vi "Parse NT Data.vi"(10 "Cluster":T1, 11 "TCP Network Connection in":refnum<k5>) -> (1 "Size":i32, 3 "Field Value Out":T2)   [LabVIEW 2017]
uses:
  <vilib>/Rock Robotics/Network Tables/Field Data.ctl
  <vilib>/Rock Robotics/Network Tables/Field Type.ctl
  <vilib>/Rock Robotics/Network Tables/Sequence.ctl
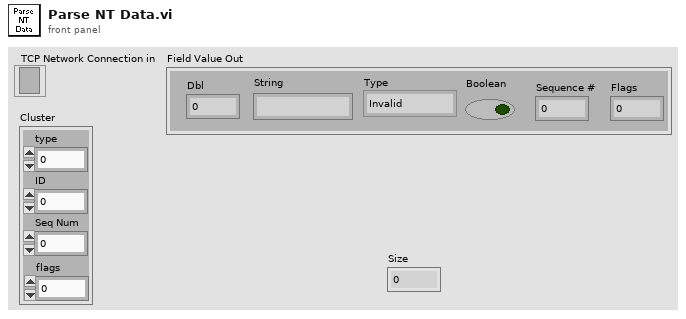
[diagram p1: front panel]
types:
  T1 = cluster{"type":u8, "ID":u16, "Seq Num":u16, "flags":u8}
  T2 = typedef "Field Data.ctl" = cluster{"Dbl":dbl, "String":string, "Type":T3, "Boolean":bool, "Sequence #":T4, "Flags":u8}
  T3 = typedef "Field Type.ctl" = enum8{"Invalid", "Bool", "Numeric", "String", "Raw", "Boolean Array", "Numeric Array", "String Array", "RPC"}
  T4 = typedef "Sequence.ctl" = u16
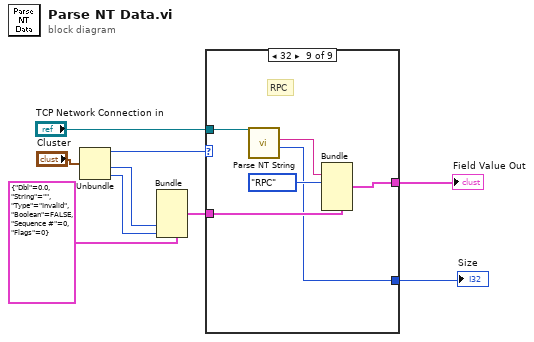
[diagram p0: block diagram]
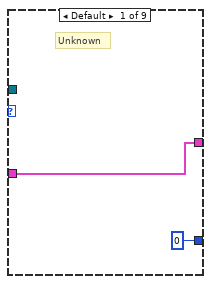
[diagram p2: hidden frame]
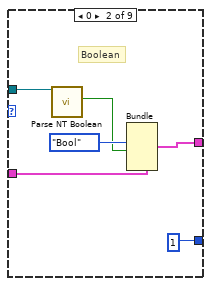
[diagram p3: hidden frame]
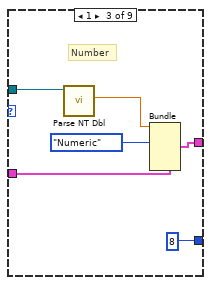
[diagram p4: hidden frame]
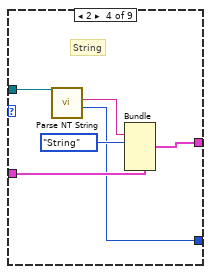
[diagram p5: hidden frame]
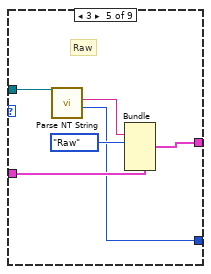
[diagram p6: hidden frame]
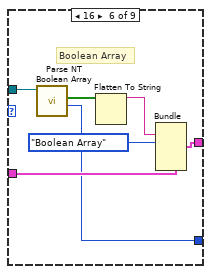
[diagram p7: hidden frame]
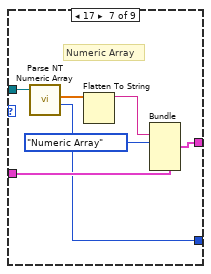
[diagram p8: hidden frame]
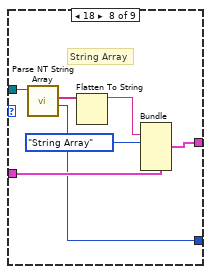
[diagram p9: hidden frame]
diagram:
  n1 = Unbundle("Cluster") -> ("type"=w7:u8, "Seq Num"=w3:u16, "flags"=w1:u8)  [unwired: 1 out]
  n2 = Bundle(cluster=T2 {"Dbl"=0.0, "String"="", "Type"=enum."Invalid", "Boolean"=FALSE, "Sequence #"=0, "Flags"=0} ("Field Value Out"), "Sequence #"=w3, "Flags"=w1) -> (w4:T2)  [unwired: 4 in]
  n3 = case shown="32" w7 {
    tunnel: "TCP Network Connection in" -> [_ w17 w23 w29 w35 w42 w49 w56 w62]
    tunnel: w4 -> [w11 w16 w21 w27 w33 w40 w47 w54 w60]
    tunnel: [w11 w13 w19 w25 w31 w39 w46 w53 w58] -> w9
    tunnel: [0 1 8 w24 w30 w36 w43 w50 w57] -> w2
    frame Default {
      # "Unknown"
    }
    frame 0 {
      # "Boolean"
      n4 = call <vilib>:"Parse NT Boolean.vi"("TCP Network Connection in"=w17) -> ("Boolean"=w14:bool)  [unwired: 9 in, 1 out]
      n5 = Bundle(cluster=w16, "Type"=Field_Type."Bool", "Boolean"=w14) -> (w13:T2)  [unwired: 4 in]
    }
    frame 1 {
      # "Number"
      n6 = call <vilib>:"Parse NT Dbl.vi"("TCP Network Connection in"=w23) -> ("Double"=w20:dbl)  [unwired: 9 in, 1 out]
      n7 = Bundle(cluster=w21, "Dbl"=w20, "Type"=Field_Type."Numeric") -> (w19:T2)  [unwired: 4 in]
    }
    frame 2 {
      # "String"
      n8 = call <vilib>:"Parse NT String.vi"("TCP Network Connection in"=w29) -> ("Size"=w24:i32, "String"=w26:string)  [unwired: 8 in, 1 out]
      n9 = Bundle(cluster=w27, "String"=w26, "Type"=Field_Type."String") -> (w25:T2)  [unwired: 4 in]
    }
    frame 3 {
      # "Raw"
      n10 = call <vilib>:"Parse NT String.vi"("TCP Network Connection in"=w35) -> ("Size"=w30:i32, "String"=w32:string)  [unwired: 8 in, 1 out]
      n11 = Bundle(cluster=w33, "String"=w32, "Type"=Field_Type."Raw") -> (w31:T2)  [unwired: 4 in]
    }
    frame 16 {
      # "Boolean Array"
      n12 = call <vilib>:"Parse NT Boolean Array.vi"("TCP Network Connection in"=w42) -> ("Size"=w36:i32, "Boolean Array"=w38:bool[])  [unwired: 7 in, 2 out]
      n13 = Flatten To String(anything=w38) -> (data string=w37:string)  [unwired: 3 in, 2 out]
      n14 = Bundle(cluster=w40, "String"=w37, "Type"=Field_Type."Boolean Array") -> (w39:T2)  [unwired: 4 in]
    }
    frame 17 {
      # "Numeric Array"
      n15 = call <vilib>:"Parse NT Numeric Array.vi"("TCP Network Connection in"=w49) -> ("Size"=w43:i32, "Numeric Array"=w45:dbl[])  [unwired: 7 in, 2 out]
      n16 = Flatten To String(anything=w45) -> (data string=w44:string)  [unwired: 3 in, 2 out]
      n17 = Bundle(cluster=w47, "String"=w44, "Type"=Field_Type."Numeric Array") -> (w46:T2)  [unwired: 4 in]
    }
    frame 18 {
      # "String Array"
      n18 = call <vilib>:"Parse NT String Array.vi"("TCP Network Connection in"=w56) -> ("Size"=w50:i32, "String Array"=w52:string[])  [unwired: 8 in, 1 out]
      n19 = Flatten To String(anything=w52) -> (data string=w51:string)  [unwired: 3 in, 2 out]
      n20 = Bundle(cluster=w54, "String"=w51, "Type"=Field_Type."String Array") -> (w53:T2)  [unwired: 4 in]
    }
    frame 32 {
      # "RPC"
      n21 = call <vilib>:"Parse NT String.vi"("TCP Network Connection in"=w62) -> ("Size"=w57:i32, "String"=w59:string)  [unwired: 8 in, 1 out]
      n22 = Bundle(cluster=w60, "String"=w59, "Type"=Field_Type."RPC") -> (w58:T2)  [unwired: 4 in]
    }
  }
  "Field Value Out" <- w9
  "Size" <- w2
